vi "TypeDef Demo.vi"() -> ()   [LabVIEW 2014]
uses:
  Controls/Strict TypeDef.ctl
  Controls/TypeDef.ctl
panel:
  in  "自定义类型":T1
  in  "严格自定义类型":T2
  in  "自定义控件":cluster{"数值输入控件":dbl, "字符串":string}
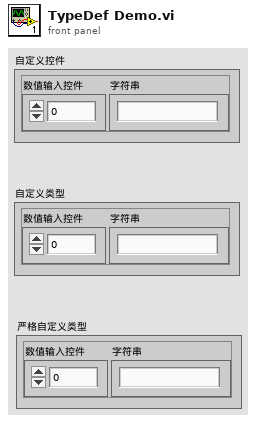
[diagram p1: front panel]
types:
  T1 = typedef "TypeDef.ctl" = cluster{"数值输入控件":dbl, "字符串":string}
  T2 = typedef "Strict TypeDef.ctl" = cluster{"数值输入控件":dbl, "字符串":string}
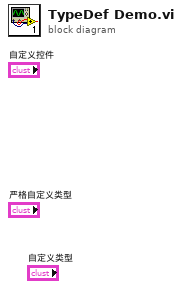
[diagram p0: block diagram]
diagram:
